vi "Options GUI.vi"(7 "Initial Tab(0)":i32, 11 "error in (no error)":errorcluster) -> (8 "OK":bool, 14 "Restart software":bool, 15 "error out":errorcluster)   [LabVIEW 2011]
uses:
  Options Page 1 for display.ctl
  Options Page 2.ctl
  Options Page 6 (Err).ctl
  Options Page 7 (Expert).ctl
  GUI/Options/Modem simulation setup.ctl
  Options Page 3.ctl
  PCP interface/PCP type List.ctl
  PCP interface/PSU Type.ctl
  Options Page 4.ctl
  Tool/Stroke force selector.ctl
  Tool/Default anchor behavior.ctl
  Tool/Default stroker behavior.ctl
  GUI/Controls/Slips Type Radio.ctl
  Options Page 5.ctl
  Options Page 8 (Depth).ctl
  Action GFV Settings.ctl
  Options PageID.ctl
  <vilib>/Utility/libraryn.llb/Check if File or Folder Exists.vi
panel:
  in  "Help":bool
  in  "Create system report":bool
  in  "Cancel":bool
  in  "OK btn":bool
  in  "Tab Control":T1(tab)
  in  "Modem Status":u16(ring) items=["Select Port", "COM19", "Refresh"]
  in  "Tractor Interface":u16(ring) items=["Select Port", "COM19", "Refresh"]
  in  "Modem Data":u16(ring) items=["Select Port", "COM19", "Refresh"]
  in  "Power Supply/PCP":u16(ring) items=["Select Port", "COM19", "Refresh"]
  in  "P 1 (App)":T2
  in  "Power supply connected":string
  in  "P 3":T3={"Min resistance"=40.0, "Max resistance"=70.0, "Head voltage range"=enum."0 - 450V", "Max voltage jump"=10.0, "Maximum resistance change"=2.0, "Start Telemetry Voltage"=35.0, "Start Telemetry Timeout"=20.0, "Start Motor Voltage"=160.0, "Stop Motor Voltage"=1.0, "Pass Mode Warning Voltage"=1.0, "Relay Switch Voltage"=160.0, "Relay Status Loss Voltage"=0.0, "Samples to average"=1, "PSU type DO NOT USE"=enum."Magna 8.3A", "Magna OVP"=1.0, "Magna Current Limit"=160.0} {"Relay Status Loss Voltage" min=0.0 max=500.0 format="%#.0f"; "Relay Switch Voltage" min=5.0 max=500.0 format="%#.0f"; "Magna Current Limit" min=0.0 max=20.0 format="%.1f"; "Magna OVP" min=0.0 max=1500.0 format="%#.0f"; "Pass Mode Warning Voltage" min=5.0 max=500.0 format="%#.0f"; "Stop Motor Voltage" min=5.0 max=500.0 format="%#.0f"; "Start Telemetry Timeout" min=0.0 max=500.0 format="%#.0f"; "Samples to average" min=1 max=10; "Start Motor Voltage" min=5.0 max=500.0 format="%#.0f"; "Start Telemetry Voltage" min=5.0 max=500.0 format="%#.0f"; "Maximum resistance change" min=1.0 max=100.0 format="%#.0f"; "Max voltage jump" min=5.0 max=500.0 format="%#.0f"; "Max resistance" min=30.0 max=500.0 format="%#.0f"; "Min resistance" min=0.0 max=500.0 format="%#.0f"}
  out "Force Unit 2":string
  out "Force Unit":string
  in  "P 4":T6={"Solenoid & Relay latching time"=40, "Stroker relay 1"=1.0, "Stroker Relay 2"=40.0, "Stroker Solenoid limit"=0.0, "Force det."=enum."Stroke in = node 1", "Stroke force lim."=0.0, "Anchor Enabled Pressure"=0.05, "Tacometer puls"=0.3, "Default anchor behavior"=enum."Do nothing", "Default stroker behavior"=enum."Do nothing", "Default stroker force limit (tonne)"=0.0, "Slips Size"=enum."338 MRS"} {"Default stroker force limit (tonne)" format="%.2f"; "Stroker Relay 2" format="%.2f"; "Stroker relay 1" format="%.2f"; "Tacometer puls" format="%.2f"; "Anchor Enabled Pressure" format="%.2f"; "Stroke force lim." format="%.2f"; "Stroker Solenoid limit" format="%.2f"}
  in  "P 5":T11={"Solenoid & Relay latching time"=0, "Driller relay 1"=0.3, "Driller Relay 2"=0.2, "Driller  Solenoid limit"=0.2} {"Driller  Solenoid limit" format="%.2f"; "Driller Relay 2" format="%.2f"; "Driller relay 1" format="%.2f"}
  in  "P 2":T12={"Solenoid & Relay latching time"=0, "Tractor relay 1"=0.3, "Tractor relay 2"=0.2, "Tractor Solenoid limit"=0.2} {"Tractor Solenoid limit" format="%.2f"; "Tractor relay 2" format="%.2f"; "Tractor relay 1" format="%.2f"}
  in  "P 6 (Err)":T13
  in  "P 7 (Expert)":T14={"Show Debug"=FALSE, "Log debug messages"=FALSE, "Additional debug messages"=FALSE, "Start Beagle with Simulator data"=FALSE, "Workshop mode"=FALSE, "Modem baud"=38400, "enumCANCOM"=FALSE, "Modem sim"={"Modem dealay sim"=FALSE, "Sim baud Tx"=1200, "Bit Error fraction Tx"=0.0, "Sim baud Rx"=1200, "Bit Error fraction Rx"=0.0}, "Telemetry Timeout Disable"=20, "Buffer size"=20, "Upd regular data"=FALSE, "Cable comp"={"VMOD1 Voltage(V)"=1.0, "VMOD2 Voltage(V)"=8.0}} {"Cable comp"."VMOD2 Voltage(V)" format="%.1f"; "Cable comp"."VMOD1 Voltage(V)" format="%.1f"; "Telemetry Timeout Disable" min=2 max=20 step=2; "Modem baud" items=["38400 (Normal use)"=38400, "9600 (Development)"=9600]; "Modem sim"."Bit Error fraction Rx" format="%.9f"; "Modem sim"."Sim baud Rx" items=["9600"=9600, "4800"=4800, "2400"=2400, "1200"=1200, "1000"=1000, "800"=800, "600"=600, "400"=400, "200"=200]; "Modem sim"."Bit Error fraction Tx" format="%.9f"; "Modem sim"."Sim baud Tx" items=["9600"=9600, "4800"=4800, "2400"=2400, "1200"=1200, "1000"=1000, "800"=800, "600"=600, "400"=400, "200"=200]; "Buffer size" min=86400 max=1209600}
  in  "Set current depth":bool caption="Solonoid 3 off"
  in  "P 8 (Depth)":T16={"Winch Spool Circumference"=100.0, "Winch Pulses per Revolution"=160.0, "Current Depth"=100.0} {"Current Depth" format="%#.7f"; "Winch Pulses per Revolution" min=1.0 max=100000.0 step=1.0 format="%#.0f"; "Winch Spool Circumference" min=0.0 max=200.0 format="%#.7f"}
  # "Tab header s can be changed as wanted\n\nCustom can be used for completly ccutom behavior,\nmust then highjack  an other hidden page, for settings"
  # "Add custom behavior taht cvan not be replicated by a simple cluster with valisdity checking"
  # "* Changes to marked options will take effect the next time you start Beagle."
  # "Ohm"
  # "Ohm"
  # "V"
  # "Ohm"
  # "V"
  # "s"
  # "V"
  # "V"
  # "V"
  # "V"
  # "V"
  # "ms"
  # "When both relays are used in \nthe same operation, the lowest\nlimit is used for both."
  # "A"
  # "A"
  # "A"
  # "Bar"
  # "ms"
  # "When both relays are used in \nthe same operation, the lowest\nlimit is used for both."
  # "A"
  # "A"
  # "A"
  # "ms"
  # "When both relays are used in \nthe same operation, the lowest\nlimit is used for both."
  # "A"
  # "A"
  # "A"
  # "Add custom behavior taht cvan not be replicated by a simple cluster with valisdity checking"
  # "Hide this page, remove this button\nAdd custom behavior if needed, using this excample"
  # "Add custom behavior taht cvan not be replicated by a simple cluster with valisdity checking"
  # "m"
  # "Pulses"
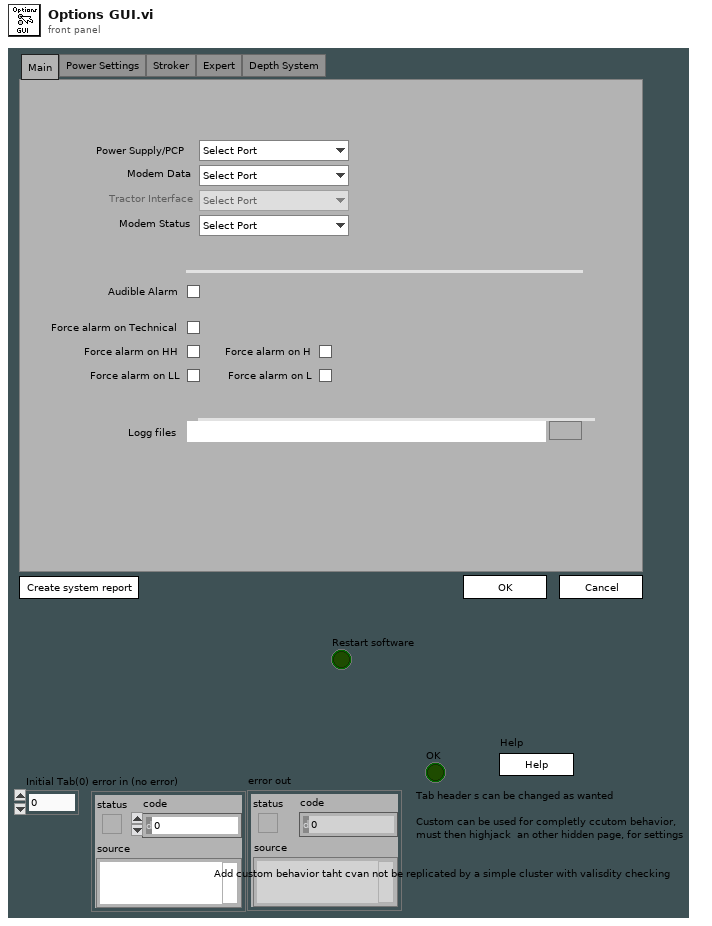
[diagram p1: front panel]
types:
  T1 = enum32{"Main", "Power Settings", "Stroker", "Driller", "Tractor", "Custom 1", "Custom 2", "Error and Events", "Expert", "Depth System"}
  T2 = typedef "Options Page 1 for display.ctl" = cluster{"Logg files":path, "Audible Alarm":bool, "Force alarm on Technical":bool, "Force alarm on HH":bool, "Force alarm on LL":bool, "Force alarm on H":bool, "Force alarm on L":bool}
  T3 = typedef "Options Page 3.ctl" = cluster{"Min resistance":dbl, "Max resistance":dbl, "Head voltage range":T4, "Max voltage jump":dbl, "Maximum resistance change":dbl, "Start Telemetry Voltage":dbl, "Start Telemetry Timeout":dbl, "Start Motor Voltage":dbl, "Stop Motor Voltage":dbl, "Pass Mode Warning Voltage":dbl, "Relay Switch Voltage":dbl, "Relay Status Loss Voltage":dbl, "Samples to average":i32, "PSU type DO NOT USE":T5, "Magna OVP":dbl, "Magna Current Limit":dbl}
  T4 = typedef "PCP type List.ctl" = enum16{"0 - 350V", "0 - 450V", "0 - 600V"}
  T5 = typedef "PSU Type.ctl" = enum16{"Unipower", "Magna 8.3A", "Magna 12A", "None"}
  T6 = typedef "Options Page 4.ctl" = cluster{"Solenoid & Relay latching time":u16, "Stroker relay 1":dbl, "Stroker Relay 2":dbl, "Stroker Solenoid limit":dbl, "Force det.":T7, "Stroke force lim.":dbl, "Anchor Enabled Pressure":dbl, "Tacometer puls":dbl, "Default anchor behavior":T8, "Default stroker behavior":T9, "Default stroker force limit (tonne)":dbl, "Slips Size":T10}
  T7 = typedef "Stroke force selector.ctl" = enum16{"Stroke in = node 1", "Strok out = node 1"}
  T8 = typedef "Default anchor behavior.ctl" = enum16{"Do nothing", "Set Anchor", "Release Anchor"}
  T9 = typedef "Default stroker behavior.ctl" = enum16{"Do nothing", "Stop", "Go Out", "Go In"}
  T10 = typedef "Slips Type Radio.ctl" = enum32{"No Selection", "338 MRS", "3,9 MRS"}
  T11 = typedef "Options Page 5.ctl" = cluster{"Solenoid & Relay latching time":u16, "Driller relay 1":dbl, "Driller Relay 2":dbl, "Driller  Solenoid limit":dbl}
  T12 = typedef "Options Page 2.ctl" = cluster{"Solenoid & Relay latching time":u16, "Tractor relay 1":dbl, "Tractor relay 2":dbl, "Tractor Solenoid limit":dbl}
  T13 = typedef "Options Page 6 (Err).ctl" = cluster{"Error and event files":path}
  T14 = typedef "Options Page 7 (Expert).ctl" = cluster{"Show Debug":bool, "Log debug messages":bool, "Additional debug messages":bool, "Start Beagle with Simulator data":bool, "Workshop mode":bool, "Modem baud":u16, "enumCANCOM":bool, "Modem sim":T15, "Telemetry Timeout Disable":i32, "Buffer size":i32, "Upd regular data":bool, "Cable comp":cluster{"VMOD1 Voltage(V)":dbl, "VMOD2 Voltage(V)":dbl}}
  T15 = typedef "Modem simulation setup.ctl" = cluster{"Modem dealay sim":bool, "Sim baud Tx":u16, "Bit Error fraction Tx":dbl, "Sim baud Rx":u16, "Bit Error fraction Rx":dbl}
  T16 = typedef "Options Page 8 (Depth).ctl" = cluster{"Winch Spool Circumference":dbl, "Winch Pulses per Revolution":dbl, "Current Depth":dbl}
  T17 = typedef "Action GFV Settings.ctl" = enum16{"Init", "Get From INI", "Put In INI", "Get Settings", "Get Update Index", "Set Setting"}
  T18 = typedef "Options  All pages and custom.ctl" = cluster{"P 1 (App)":T19, "P 2":T12, "P 3":T3, "P 4":T6, "P 5":T11, "P 6 (Err)":T13, "P 7 (Expert)":T14, "P 8 (Depth)":T16, "C 1":T20, "C 2":T21}
  T19 = typedef "Options Page 1 (App).ctl" = cluster{"Result files":path, "PCP Interface":string, "Tractor/Stroker Interface":string, "Tractor Interface":string, "Modem Status Interface":string, "Audible Alarm":bool, "Force alarm on Technical":bool, "Force alarm on HH":bool, "Force alarm on LL":bool, "Force alarm on H":bool, "Force alarm on L":bool}
  T20 = typedef "Options Custom 1.ctl" = cluster{"Depth Updated":bool, "Depth Offset":dbl}
  T21 = typedef "Options Custom 2.ctl" = cluster{"Placeholder":bool}
  T22 = enum8{"Enabled", "Disabled", "Disabled and Grayed Out"}
  T23 = typedef "List of tools.ctl" = enum16{"Stroker", "Driller", "Tractor"}
  T24 = typedef "User Indikator.ctl" = cluster{"User Name":string, "Super User":T25}
  T25 = typedef "Super User bool indikator.ctl" = bool
  T26 = typedef "Options PageID.ctl" = enum16{"P 1 (App)", "P 2", "P 3", "P 4", "P 5", "P 6 (Err)", "P 7 (Expert)", "P 8", "C 1", "C 2"}
  T27 = enum16{"open", "replace", "create", "open or create", "replace or create", "replace or create with confirmation"}
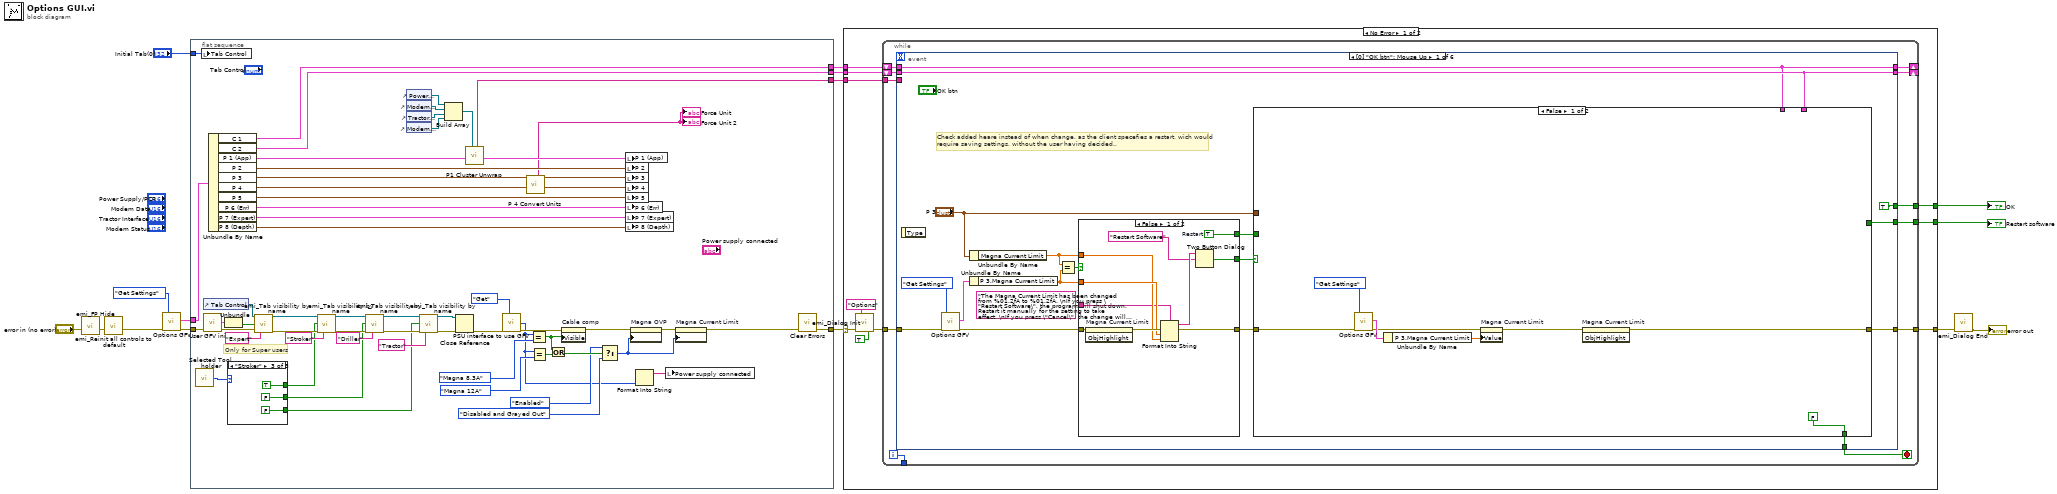
[diagram p0: block diagram]
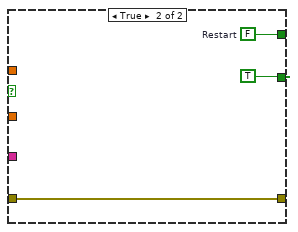
[diagram p2: hidden frame]
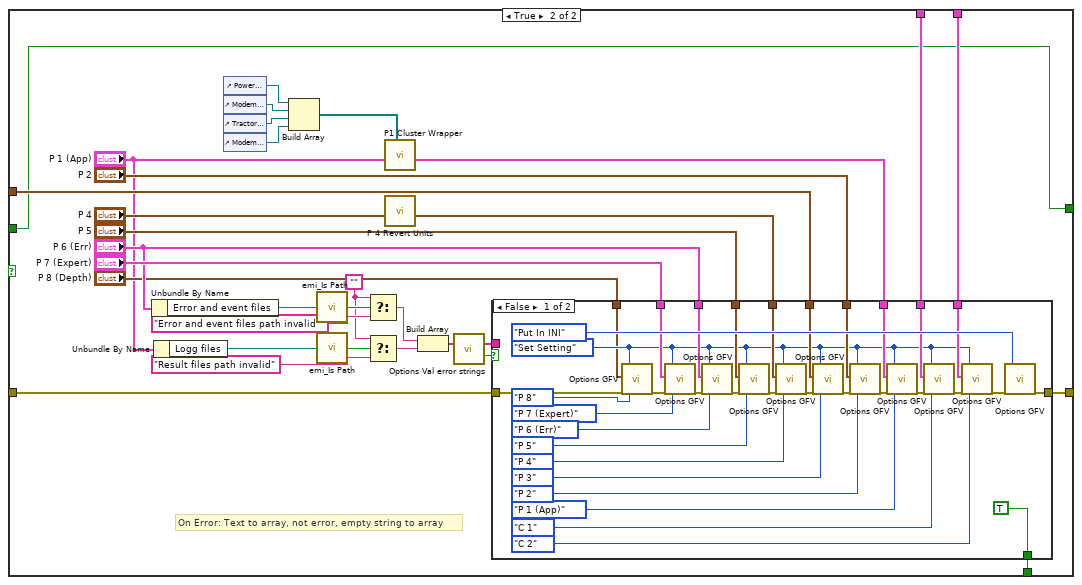
[diagram p3: hidden frame]
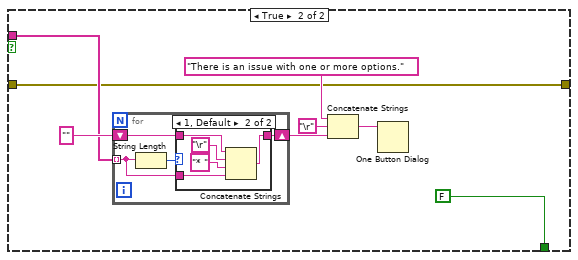
[diagram p4: hidden frame]
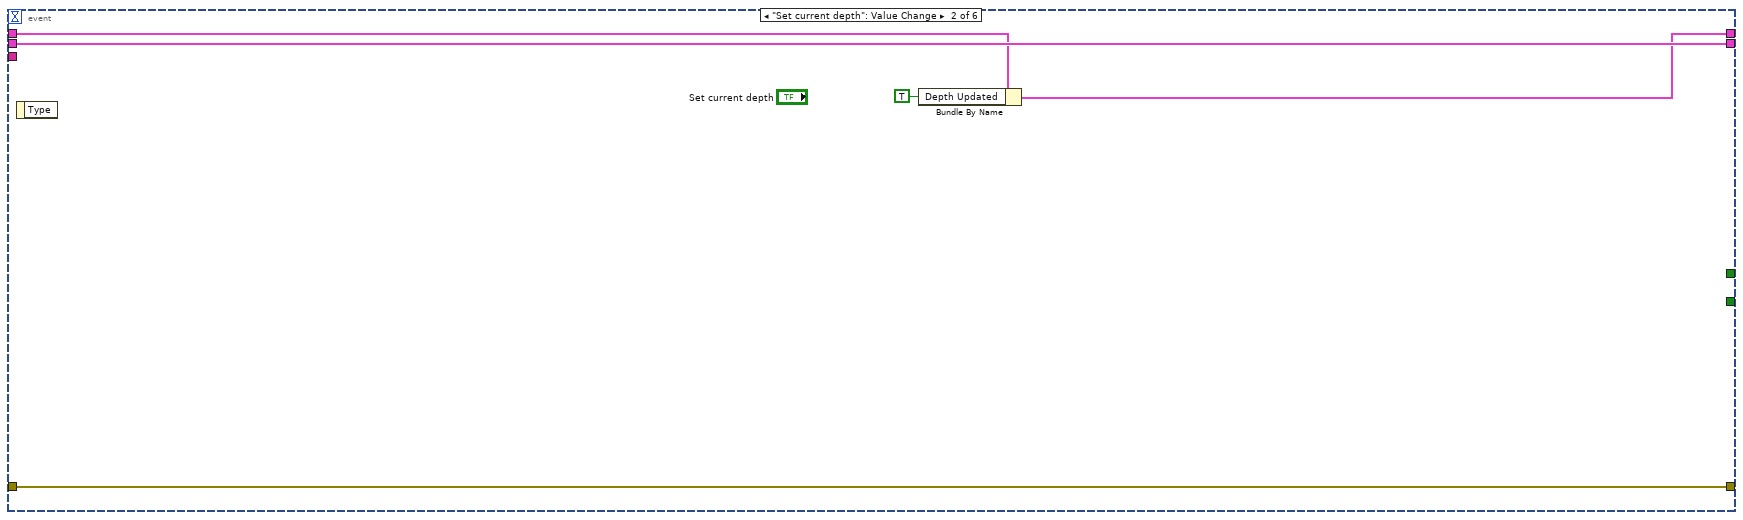
[diagram p6: hidden frame]
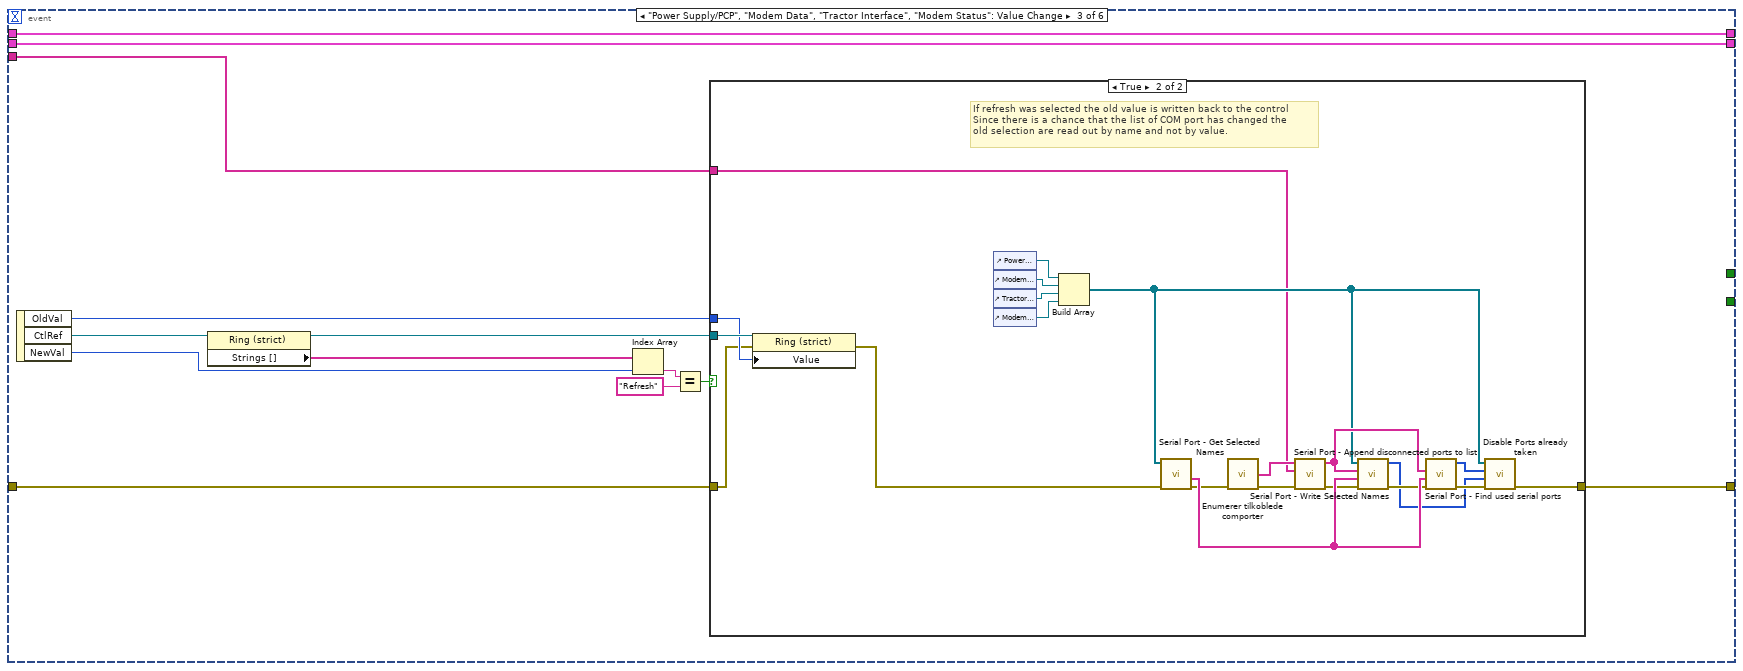
[diagram p7: hidden frame]
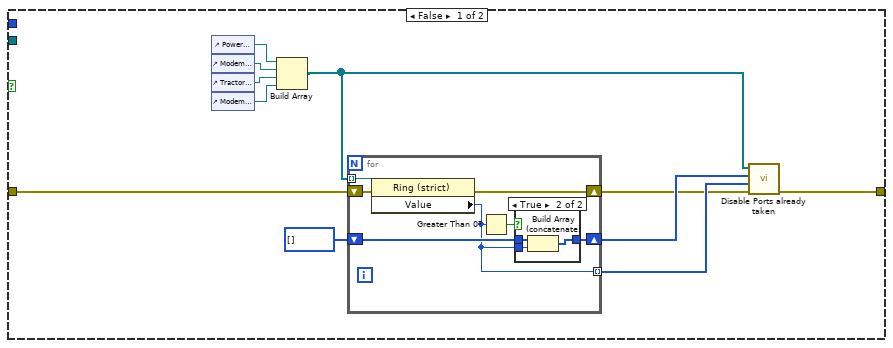
[diagram p8: hidden frame]
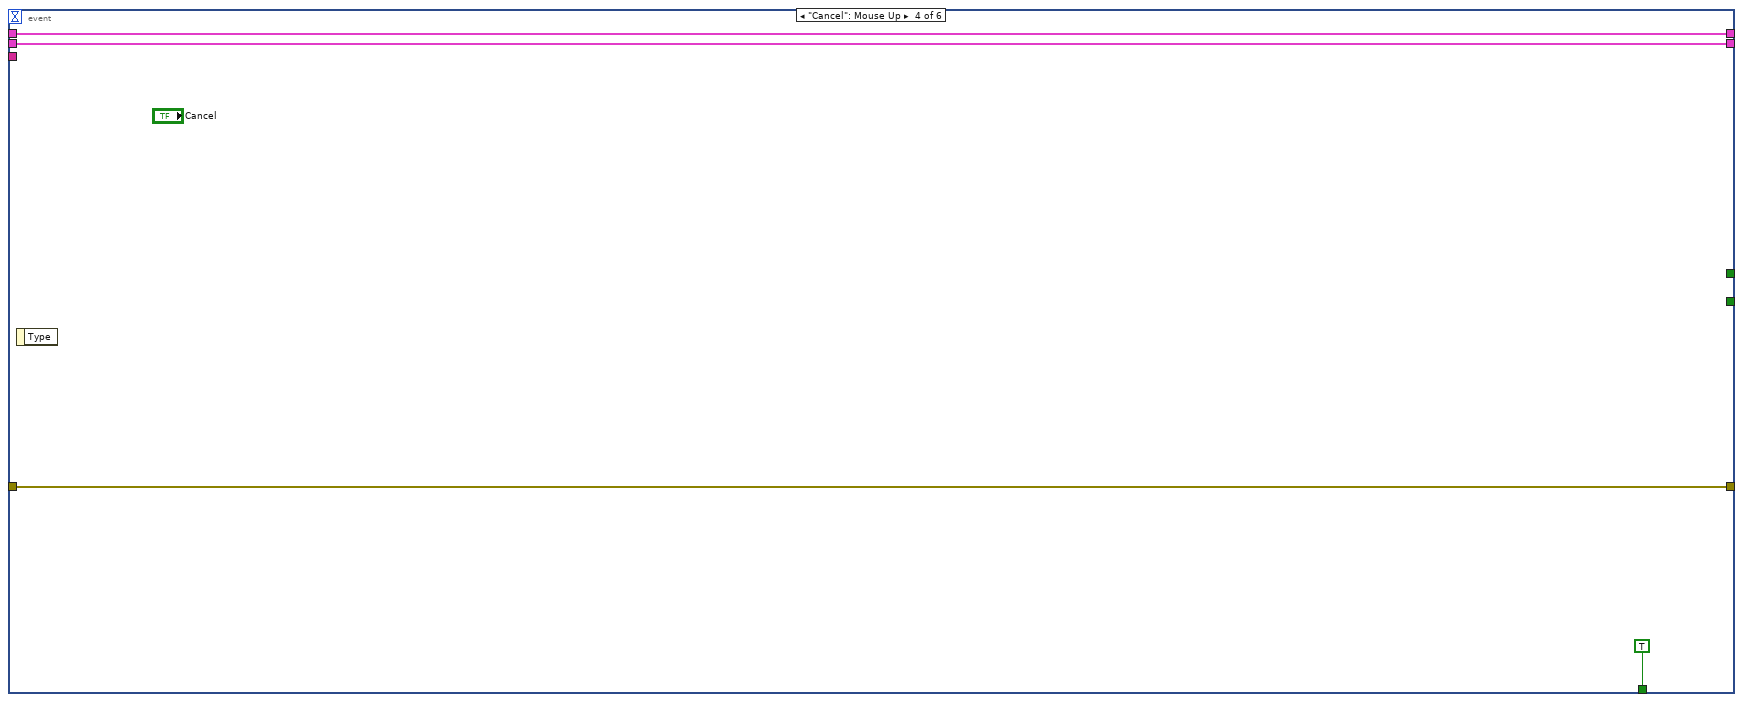
[diagram p10: hidden frame]
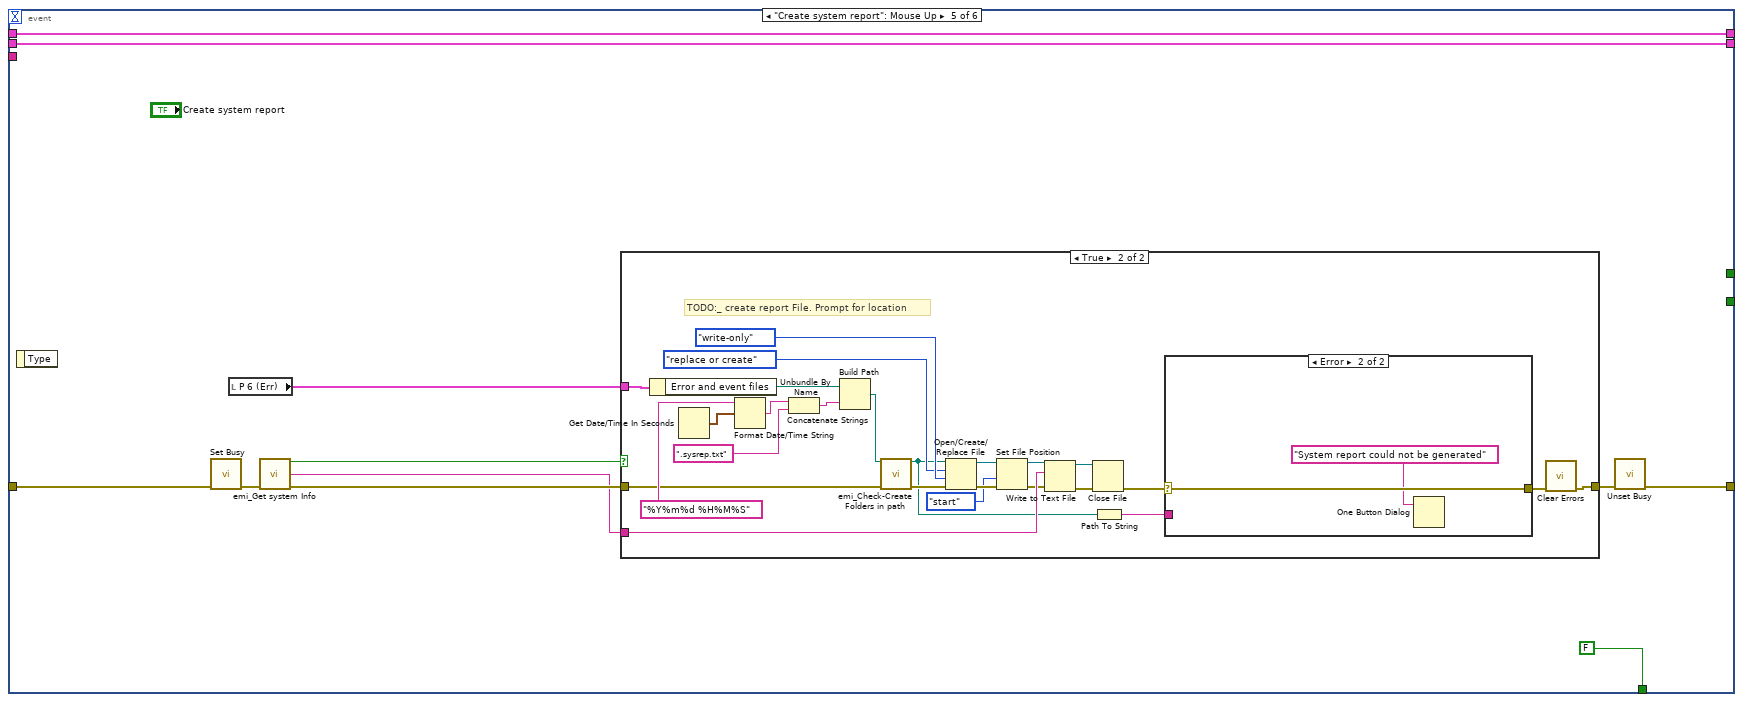
[diagram p11: hidden frame]
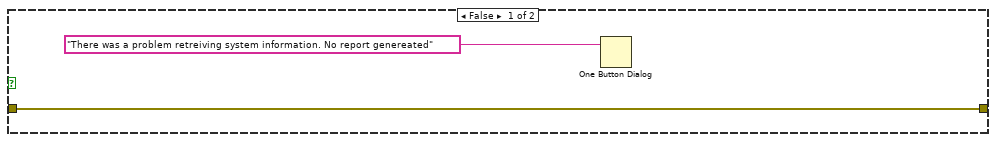
[diagram p12: hidden frame]
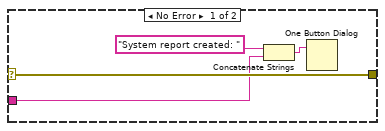
[diagram p13: hidden frame]
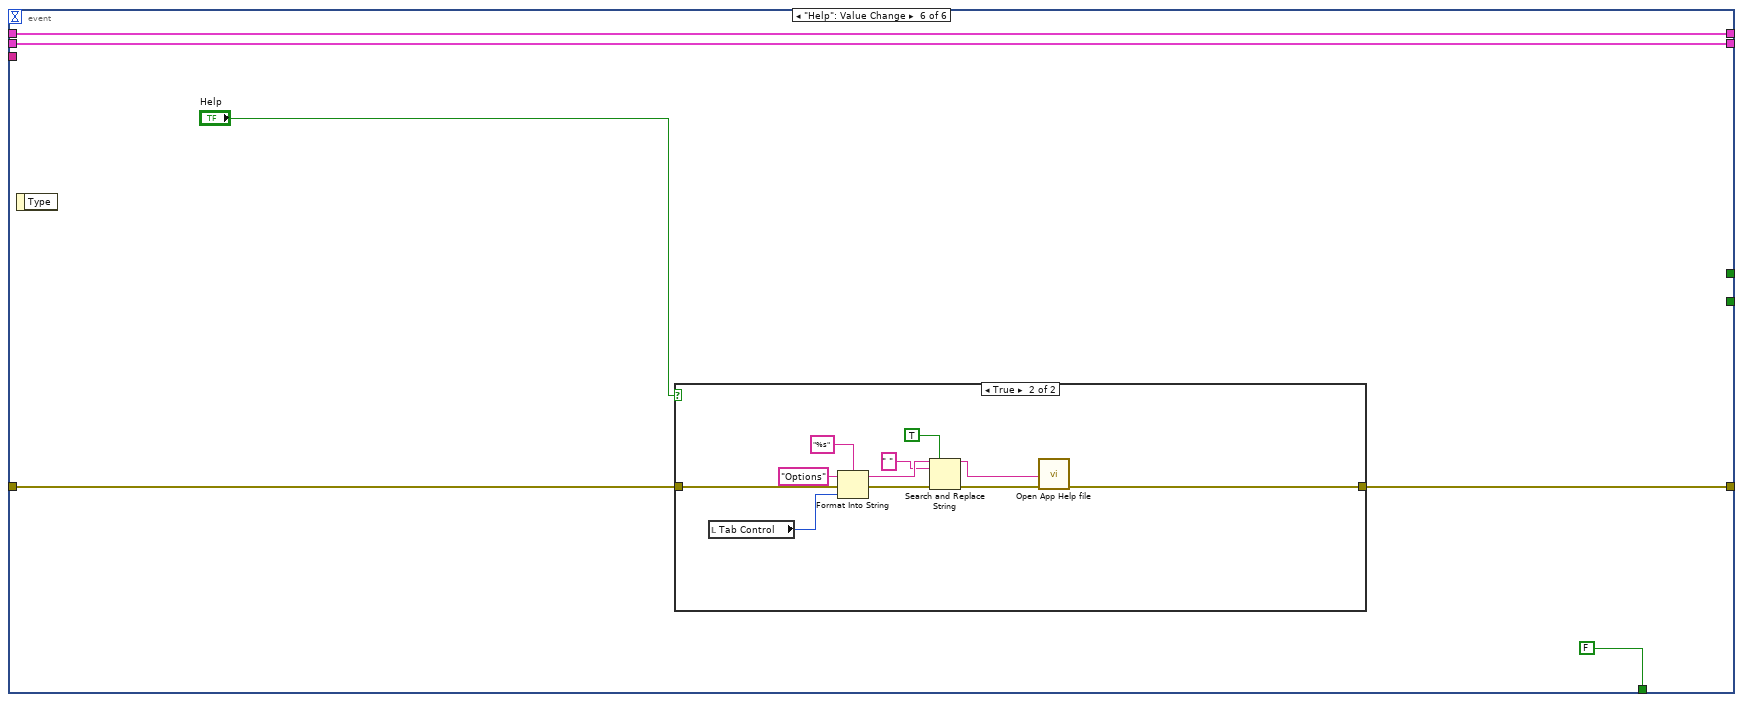
[diagram p14: hidden frame]
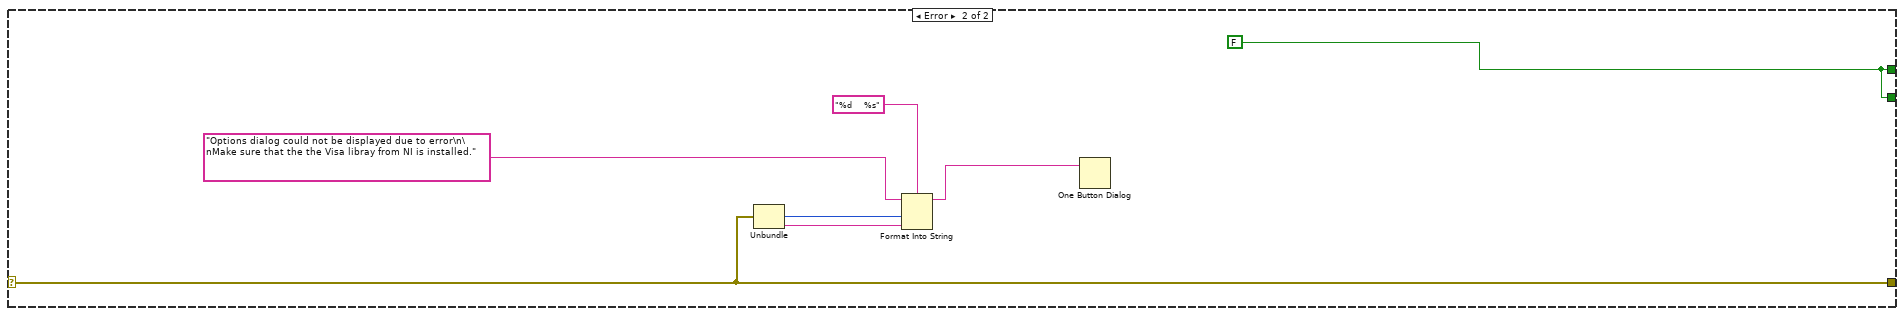
[diagram p16: hidden frame]
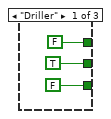
[diagram p17: hidden frame]
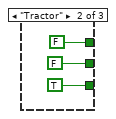
[diagram p18: hidden frame]
diagram:
  n1 = call "emi_FP Hide.vi"("error in (no error)"="error in (no error)") -> ("error out"=w5:errorcluster)  [unwired: 13 in, 1 out]
  n2 = call "emi_Reinit all controls to default.vi"("error in (no error)"=w5) -> ("error out"=w4:errorcluster)  [unwired: 13 in, 1 out]
  n3 = call "Options GFV.vi"("error in (no error)"=w4, "Action(Get Settings)"=Action_GFV_Settings."Get Settings" ("Action")) -> ("Options"=w12:T18, "error out"=w13:errorcluster)  [unwired: 15 in, 1 out]
  n4 = flat-sequence {
    tunnel: [w28] -> w3
    tunnel: "Initial Tab(0)" -> [w70]
    tunnel: w13 -> [w68]
    tunnel: w12 -> [w69]
    tunnel: [w45] -> w9
    tunnel: [w46] -> w10
    tunnel: [w33] -> w2
    frame #0 {
      # "Only for Super users"
      n5 = call "Selected Tool holder.vi"() -> ("Tool out"=w51:T23)  [unwired: 14 in, 1 out]
      n6 = local write "Tab Control"(w70) -> ()
      n7 = control-ref of="Tab Control"() -> (w65:refnum<vi>)
      n8 = call "User GFV ini.vi"("error in (no error)"=w68) -> ("User ID out"=w67:T24, "error out"=w66:errorcluster)  [unwired: 13 in]
      n9 = Unbundle By Name(w69) -> ("C 1"=w46:T20, "C 2"=w45:T21, "P 1 (App)"=w36:T19, "P 2"=w74:T12, "P 3"=w73:T3, "P 4"=w43:T6, "P 5"=w47:T11, "P 6 (Err)"=w72:T13, "P 7 (Expert)"=w71:T14, "P 8 (Depth)"=w44:T16)
      n10 = Unbundle(w67) -> ("Super User"=w64:T25)  [unwired: 1 out]
      n11 = case shown="\"Stroker\"" w51 {
        tunnel: [FALSE ("Visibil(T)") FALSE ("Visibil(T)") TRUE ("Visibil(T)")] -> w50
        tunnel: [TRUE ("Visibil(T)") FALSE ("Visibil(T)") FALSE ("Visibil(T)")] -> w49
        tunnel: [FALSE ("Visibil(T)") TRUE ("Visibil(T)") FALSE ("Visibil(T)")] -> w48
        frame "Driller" {
        }
        frame "Tractor" {
        }
        frame "Stroker" {
        }
      }
      n12 = call "emi_Tab visibility by name.vi"("reference"=w65, "Visibil(T)"=w64, "error in (no error)"=w66, "Tab name(\"Debug\")"="Expert" ("Tab name(\"Debug\")")) -> ("reference out"=w61:refnum<vi>, "error out"=w62:errorcluster)  [unwired: 10 in]
      n13 = call "emi_Tab visibility by name.vi"("reference"=w61, "Visibil(T)"=w50, "error in (no error)"=w62, "Tab name(\"Debug\")"="Stroker" ("Tab name(\"Debug\")")) -> ("reference out"=w59:refnum<vi>, "error out"=w60:errorcluster)  [unwired: 10 in]
      n14 = call "emi_Tab visibility by name.vi"("reference"=w59, "Visibil(T)"=w49, "error in (no error)"=w60, "Tab name(\"Debug\")"="Driller" ("Tab name(\"Debug\")")) -> ("reference out"=w57:refnum<vi>, "error out"=w58:errorcluster)  [unwired: 10 in]
      n15 = control-ref of="Power Supply/PCP"() -> (w41:refnum<vi>)
      n16 = control-ref of="Modem Data"() -> (w40:refnum<vi>)
      n17 = control-ref of="Tractor Interface"() -> (w39:refnum<vi>)
      n18 = control-ref of="Modem Status"() -> (w38:refnum<vi>)
      n19 = call "emi_Tab visibility by name.vi"("reference"=w57, "Visibil(T)"=w48, "error in (no error)"=w58, "Tab name(\"Debug\")"="Tractor" ("Tab name(\"Debug\")")) -> ("reference out"=w55:refnum<vi>, "error out"=w56:errorcluster)  [unwired: 10 in]
      n20 = Build Array(w41, w40, w39, w38) -> (w35:refnum<vi>[])
      n21 = Close Reference(reference=w55, error in (no error)=w56) -> (error out=w32:errorcluster)
      n22 = call "P1 Cluster Unwrap.vi"("COM Selector Refs"=w35, "P 1 (App) in"=w36) -> ("P 1 (App) out"=w37:T2, "Initial selection"=w33:string[])  [unwired: 8 in]
      n23 = call "PSU interface to use GFV.vi"("Action"=enum16{"Get", "Set"}."Get", "error in (no error)"=w32) -> ("PSU type  out"=w17:T5, "error out"=w30:errorcluster)  [unwired: 12 in]
      n24 = call "P 4 Convert Units.vi"("P 4"=w43) -> ("P 4"=w42:T6, "Unit"=→"Force Unit" →"Force Unit 2":string)  [unwired: 9 in]
      n25 = Equal?(x=w17, y=PSU_Type."Magna 8.3A") -> (x = y?=w25:bool)
      n26 = Equal?(x=w17, y=PSU_Type."Magna 12A") -> (x = y?=w26:bool)
      n27 = Or(x=w25, y=w26) -> (x .or. y?=w21:bool)
      n28 = property on="Cable comp" class="Clust (strict)"(error in=w30, "Visible"=w25) -> (error out=w24:errorcluster)  [unwired: 1 in, 1 out]
      n29 = Select(t=T22."Enabled" ("Disabled"), s=w21, f=T22."Disabled and Grayed Out" ("Disabled")) -> (s? t:f=w18:T22)
      n30 = local write "P 1 (App)"(w37) -> ()
      n31 = local write "P 2"(w74) -> ()
      n32 = local write "P 3"(w73) -> ()
      n33 = local write "P 4"(w42) -> ()
      n34 = local write "P 5"(w47) -> ()
      n35 = local write "P 6 (Err)"(w72) -> ()
      n36 = local write "P 7 (Expert)"(w71) -> ()
      n37 = local write "P 8 (Depth)"(w44) -> ()
      n38 = property on="Magna OVP" class="DigNum (strict)"(error in=w24, "DisabledEnum"=w18) -> (error out=w23:errorcluster)  [unwired: 1 in, 1 out]
      n39 = Format Into String(w17) -> (resulting string=w16:string)  [unwired: 3 in, 1 out]
      n40 = local write "Power supply connected"(w16) -> ()
      n41 = property on="Magna Current Limit" class="DigNum (strict)"(error in=w23, "DisabledEnum"=w18) -> (error out=w22:errorcluster)  [unwired: 1 in, 1 out]
      n42 = call <vilib>:"Clear Errors.vi"("error in (no error)"=w22) -> ("error out"=w28:errorcluster)  [unwired: 6 in]
    }
  }
  n43 = case shown="No Error" w3 {
    selector: w3 -> [w86 w363]
    tunnel: w10 -> [w93 _]
    tunnel: w9 -> [w92 _]
    tunnel: [w91 w357] -> w8
    tunnel: [w90 w363] -> w7
    tunnel: w2 -> [w85 _]
    tunnel: [w84 w357] -> w1
    frame No Error {
      n44 = call "emi_Dialog Init.vi"("Header String(\"\")"="Options" ("Header String(\"\")"), "error in"=w86, "Modal(T)"=TRUE) -> ("error out"=w89:errorcluster)  [unwired: 12 in]
      n45 = while {
        tunnel: [w104] -> _
        tunnel: w89 -> [w103]
        tunnel: [w102] -> w90
        shift-right: [w99] -> _
        shift-left: w93 -> [w101]
        shift-right: [w98] -> _
        shift-left: w92 -> [w100]
        tunnel: [w97] -> w91
        tunnel: w85 -> [w95]
        tunnel: [w94] -> w84
        i -> [w104]
        stop <- w96 stop-if-true
        n46 = event shown="[0] \"OK btn\": Mouse Up" {
          selector: _ -> [_ _ _ _ _ _]
          dyn-events: _ -> [_ _ _ _ _ _]
          timeout: _ -> [_ _ _ _ _ _]
          tunnel: [w122 _ _ TRUE FALSE FALSE] -> w96
          tunnel: w103 -> [w117 w234 w245 w293 w304 w340]
          tunnel: [w121 w234 w244 w293 w303 w341] -> w102
          tunnel: w101 -> [w118 w232 w247 w292 w296 w343]
          tunnel: w100 -> [w120 w233 w246 w291 w295 w342]
          tunnel: [w118 w231 w247 w292 w296 w343] -> w99
          tunnel: [w120 w233 w246 w291 w295 w342] -> w98
          tunnel: [TRUE _ _ _ _ _] -> w97
          tunnel: w95 -> [_ _ w235 _ _ _]
          tunnel: [w105 _ _ _ _ _] -> w94
          event "OK btn": Mouse Up {
            # "Check added heare instead of when change, as the client specefies a restart, wich would \nrequire saving settings, without the user having decided.,"
            n47 = event-data() -> ()  [unwired: 1 in, 1 out]
            n48 = call "Options GFV.vi"("error in (no error)"=w117, "Action(Get Settings)"=Action_GFV_Settings."Get Settings") -> ("Options"=w114:T18, "error out"=w111:errorcluster)  [unwired: 15 in, 1 out]
            n49 = Unbundle By Name("P 3") -> ("Magna Current Limit"=w108:dbl)
            n50 = Unbundle By Name(w114) -> ("P 3.Magna Current Limit"=w109:dbl)
            n51 = Equal?(x=w108, y=w109) -> (x = y?=w113:bool)
            n52 = case shown="False" w113 {
              tunnel: [w124 TRUE] -> w112
              tunnel: w111 -> [w132 w134]
              tunnel: [w130 w134] -> w110
              tunnel: w109 -> [w129 _]
              tunnel: w108 -> [w128 _]
              tunnel: "The Magna Current Limit has been changed from %01.2fA to %01.2fA. \nIf you press \"Restart Software\", the program will shut down. Restart it manually for the setting to take effect. \nIf you press \"Cancel\", the change will be reverted." ("format string") -> [w127 _]
              tunnel: [w123 w133] -> w106
              frame False {
                w123 = TRUE  # Restart
                n53 = invoke on="Magna Current Limit" class="DigNum (strict)" method="ObjHighlight"(error in=w132) -> (error out=w131:errorcluster)  [unwired: 2 in, 2 out]
                n54 = Format Into String(format string=w127, error in=w131, w129, w128) -> (resulting string=w126:string, error out=w130:errorcluster)  [unwired: 1 in]
                n55 = Two Button Dialog(message=w126, 2:"Restart Software" ("T button name (\"OK\")")) -> (T button?=w124:bool)  [unwired: 1 in]
              }
              frame True {
                w133 = FALSE  # Restart
              }
            }
            n56 = case shown="False" w112 {
              tunnel: [FALSE w176] -> w122
              tunnel: [w136 w175] -> w121
              tunnel: "P 3" -> [_ w174]
              tunnel: w110 -> [w140 w170]
              tunnel: w120 -> [_ w156]
              tunnel: w118 -> [_ w154]
              tunnel: w106 -> [_ w144]
              tunnel: [_ w144] -> w105
              frame False {
                n57 = call "Options GFV.vi"("error in (no error)"=w140, "Action(Get Settings)"=Action_GFV_Settings."Get Settings") -> ("Options"=w142:T18, "error out"=w138:errorcluster)  [unwired: 15 in, 1 out]
                n58 = Unbundle By Name(w142) -> ("P 3.Magna Current Limit"=w139:dbl)
                n59 = property on="Magna Current Limit" class="DigNum (strict)"(error in=w138, "Value"=w139) -> (error out=w137:errorcluster)  [unwired: 1 in, 1 out]
                n60 = invoke on="Magna Current Limit" class="DigNum (strict)" method="ObjHighlight"(error in=w137) -> (error out=w136:errorcluster)  [unwired: 2 in, 2 out]
              }
              frame True {
                w160 = ""
                # "On Error: Text to array, not error, empty string to array"
                n61 = Unbundle By Name("P 6 (Err)") -> ("Error and event files"=w166:path)
                n62 = Unbundle By Name("P 1 (App)") -> ("Logg files"=w165:path)
                n63 = control-ref of="Power Supply/PCP"() -> (w146:refnum<vi>)
                n64 = control-ref of="Modem Data"() -> (w147:refnum<vi>)
                n65 = control-ref of="Tractor Interface"() -> (w148:refnum<vi>)
                n66 = control-ref of="Modem Status"() -> (w149:refnum<vi>)
                n67 = Build Array(w146, w147, w148, w149) -> (w145:refnum<vi>[])
                n68 = call "emi_Is Path.vi"("Path"=w166) -> ("Path?"=w164:bool)  [unwired: 14 in]
                n69 = call "emi_Is Path.vi"("Path"=w165) -> ("Path?"=w163:bool)  [unwired: 14 in]
                n70 = Select(t=w160, s=w164, f="Error and event files path invalid") -> (s? t:f=w158:string)
                n71 = Select(t=w160, s=w163, f="Result files path invalid") -> (s? t:f=w157:string)
                n72 = call "P1 Cluster Wrapper.vi"("COM Selector Refs"=w145, "P 1 (App) in"="P 1 (App)") -> ("P 1 (App) out"=w150:T19)  [unwired: 8 in, 1 out]
                n73 = call "P 4 Revert Units.vi"("P 4"="P 4") -> ("P 4"=w152:T6)  [unwired: 10 in]
                n74 = Build Array(w158, w157) -> (w159:string[])
                n75 = call "Options Val error strings.vi"("Array of error strings"=w159) -> ("Array of error strings out"=w171:string[], "Error"=w172:bool)  [unwired: 13 in]
                n76 = case shown="False" w172 {
                  tunnel: [TRUE FALSE] -> w176
                  tunnel: [w204 w212] -> w175
                  tunnel: w150 -> [w196 _]
                  tunnel: "P 2" -> [w195 _]
                  tunnel: w174 -> [w194 _]
                  tunnel: w152 -> [w193 _]
                  tunnel: "P 5" -> [w192 _]
                  tunnel: "P 6 (Err)" -> [w191 _]
                  tunnel: "P 7 (Expert)" -> [w190 _]
                  tunnel: w171 -> [_ w213]
                  tunnel: w170 -> [w181 w212]
                  tunnel: w156 -> [w185 _]
                  tunnel: w154 -> [w186 _]
                  tunnel: "P 8 (Depth)" -> [w177 _]
                  frame False {
                    w179 = Action_GFV_Settings."Set Setting" ("Action")
                    n77 = call "Options GFV.vi"("Anything"=w177, "error in (no error)"=w181, "Action(Get Settings)"=w179, "Setting ID"=Options_PageID."P 8") -> ("error out"=w180:errorcluster)  [unwired: 13 in, 2 out]
                    n78 = call "Options GFV.vi"("Anything"=w190, "error in (no error)"=w180, "Action(Get Settings)"=w179, "Setting ID"=Options_PageID."P 7 (Expert)") -> ("error out"=w208:errorcluster)  [unwired: 13 in, 2 out]
                    n79 = call "Options GFV.vi"("Anything"=w191, "error in (no error)"=w208, "Action(Get Settings)"=w179, "Setting ID"=Options_PageID."P 6 (Err)") -> ("error out"=w209:errorcluster)  [unwired: 13 in, 2 out]
                    n80 = call "Options GFV.vi"("Anything"=w192, "error in (no error)"=w209, "Action(Get Settings)"=w179, "Setting ID"=Options_PageID."P 5") -> ("error out"=w203:errorcluster)  [unwired: 13 in, 2 out]
                    n81 = call "Options GFV.vi"("Anything"=w193, "error in (no error)"=w203, "Action(Get Settings)"=w179, "Setting ID"=Options_PageID."P 4") -> ("error out"=w202:errorcluster)  [unwired: 13 in, 2 out]
                    n82 = call "Options GFV.vi"("Anything"=w194, "error in (no error)"=w202, "Action(Get Settings)"=w179, "Setting ID"=Options_PageID."P 3") -> ("error out"=w201:errorcluster)  [unwired: 13 in, 2 out]
                    n83 = call "Options GFV.vi"("Anything"=w195, "error in (no error)"=w201, "Action(Get Settings)"=w179, "Setting ID"=Options_PageID."P 2") -> ("error out"=w198:errorcluster)  [unwired: 13 in, 2 out]
                    n84 = call "Options GFV.vi"("Anything"=w196, "error in (no error)"=w198, "Action(Get Settings)"=w179, "Setting ID"=Options_PageID."P 1 (App)") -> ("error out"=w188:errorcluster)  [unwired: 13 in, 2 out]
                    n85 = call "Options GFV.vi"("Anything"=w186, "error in (no error)"=w188, "Action(Get Settings)"=w179, "Setting ID"=Options_PageID."C 1") -> ("error out"=w187:errorcluster)  [unwired: 13 in, 2 out]
                    n86 = call "Options GFV.vi"("Anything"=w185, "error in (no error)"=w187, "Action(Get Settings)"=w179, "Setting ID"=Options_PageID."C 2") -> ("error out"=w182:errorcluster)  [unwired: 13 in, 2 out]
                    n87 = call "Options GFV.vi"("error in (no error)"=w182, "Action(Get Settings)"=Action_GFV_Settings."Put In INI" ("Action")) -> ("error out"=w204:errorcluster)  [unwired: 15 in, 2 out]
                  }
                  frame True {
                    n88 = for {
                      shift-right: [w223] -> w215
                      shift-left: "" -> [w222]
                      tunnel: w213 -> [w220] mode=indexing
                      n89 = String Length(string=w220) -> (length=w221:i32)
                      n90 = case shown="1, Default" w221 {
                        tunnel: w222 -> [w224 w229]
                        tunnel: [w224 w226] -> w223
                        tunnel: w220 -> [_ w225]
                        frame 0 {
                        }
                        frame 1, Default {
                          n91 = Concatenate Strings(w229, "\r", "* " ("string"), w225) -> (w226:string)
                        }
                      }
                    }
                    n92 = Concatenate Strings("There is an issue with one or more options." ("message"), "\r", w215) -> (w214:string)
                    n93 = One Button Dialog(message=w214) -> ()  [unwired: 1 in, 1 out]
                  }
                }
              }
            }
          }
          event "Set current depth": Value Change {
            n94 = event-data() -> ()  [unwired: 1 in, 1 out]
            n95 = Bundle By Name(cluster=w232, "Depth Updated"=TRUE) -> (w231:T20)
          }
          event "Power Supply/PCP", "Modem Data", "Tractor Interface", "Modem Status": Value Change {
            n96 = event-data() -> ("OldVal"=w237:u16, "CtlRef"=w243:refnum<vi>, "NewVal"=w239:u16)  [unwired: 1 in]
            n97 = property class="Ring (strict)"(reference=w243) -> (reference out=w236:refnum<vi>, "Strings []"=w242:string[])  [unwired: 1 in, 1 out]
            n98 = Index Array(array=w242, index=w239) -> (element=w240:string)
            n99 = Equal?(x=w240, y="Refresh") -> (x = y?=w238:bool)
            n100 = case shown="True" w238 {
              tunnel: w245 -> [w254 w288]
              tunnel: [w253 w277] -> w244
              tunnel: w237 -> [_ w289]
              tunnel: w236 -> [_ w290]
              tunnel: w235 -> [_ w270]
              frame False {
                n101 = control-ref of="Power Supply/PCP"() -> (w249:refnum<vi>)
                n102 = control-ref of="Modem Data"() -> (w250:refnum<vi>)
                n103 = control-ref of="Tractor Interface"() -> (w251:refnum<vi>)
                n104 = control-ref of="Modem Status"() -> (w252:refnum<vi>)
                n105 = Build Array(w249, w250, w251, w252) -> (w248:refnum<vi>[])
                n106 = for {
                  tunnel: w248 -> [w265] mode=indexing
                  shift-right: [w264] -> w256
                  shift-left: w254 -> [w263]
                  tunnel: [w260] -> w258 mode=indexing
                  shift-right: [w262] -> w257
                  shift-left: i32[] [] -> [w261]
                  n107 = property class="Ring (strict)"(reference=w265, error in=w263) -> (error out=w264:errorcluster, "Value"=w260:u16)  [unwired: 1 out]
                  n108 = Greater Than 0?(x=w260) -> (x > 0?=w259:bool)
                  n109 = case shown="True" w259 {
                    tunnel: w260 -> [_ w269]
                    tunnel: [w266 w268] -> w262
                    tunnel: w261 -> [w266 w267]
                    frame False {
                    }
                    frame True {
                      n110 = Build Array (concatenate)(w267, w269) -> (w268:i32[])
                    }
                  }
                }
                n111 = call "Disable Ports already taken.vi"("error in (no error)"=w256, "Values"=w258, "COM Port numbers taken"=w257, "Ctrl References"=w248) -> ("error out"=w253:errorcluster)  [unwired: 7 in]
              }
              frame True {
                # "If refresh was selected the old value is written back to the control\nSince there is a chance that the list of COM port has changed the \nold selection are read out by name and not by value."
                n112 = property class="Ring (strict)"(reference=w290, error in=w288, "Value"=w289) -> (error out=w276:errorcluster)  [unwired: 1 out]
                n113 = control-ref of="Power Supply/PCP"() -> (w272:refnum<vi>)
                n114 = control-ref of="Modem Data"() -> (w273:refnum<vi>)
                n115 = control-ref of="Tractor Interface"() -> (w274:refnum<vi>)
                n116 = control-ref of="Modem Status"() -> (w275:refnum<vi>)
                n117 = Build Array(w272, w273, w274, w275) -> (w271:refnum<vi>[])
                n118 = call "Serial Port - Get Selected Names.vi"("error in (no error)"=w276, "Ctrl Refs in"=w271) -> ("error out"=w282:errorcluster, "Selected Names"=w287:string[])  [unwired: 8 in]
                n119 = call "Enumerer tilkoblede comporter.vi"("error in (no error)"=w282) -> ("Com port w Select string"=w281:string[], "error out"=w280:errorcluster)  [unwired: 11 in, 2 out]
                n120 = call "Serial Port - Append disconnected ports to list.vi"("error in (no error)"=w280, "Selected Values"=w270, "Connected COM Ports in"=w281) -> ("error out"=w284:errorcluster, "COM Ports out"=w283:string[])  [unwired: 7 in]
                n121 = call "Serial Port - Write Selected Names.vi"("error in (no error)"=w284, "Selected Names"=w287, "COM Port List"=w283, "Ctrl Refs in"=w271) -> ("error out"=w285:errorcluster, "Selected Values"=w278:i32[])  [unwired: 6 in]
                n122 = call "Serial Port - Find used serial ports.vi"("error in (no error)"=w285, "Selected Values"=w287, "COM Ports list"=w283) -> ("error out"=w286:errorcluster, "Items to disable"=w279:i32[])  [unwired: 7 in]
                n123 = call "Disable Ports already taken.vi"("error in (no error)"=w286, "Values"=w278, "COM Port numbers taken"=w279, "Ctrl References"=w271) -> ("error out"=w277:errorcluster)  [unwired: 7 in]
              }
            }
          }
          event "Cancel": Mouse Up {
            n124 = event-data() -> ()  [unwired: 1 in, 1 out]
          }
          event "Create system report": Mouse Up {
            n125 = event-data() -> ()  [unwired: 1 in, 1 out]
            n126 = call <vilib>:"Set Busy.vi"("error in (no error)"=w304) -> ("error out"=w302:errorcluster)  [unwired: 9 in, 1 out]
            n127 = local read "P 6 (Err)"() -> (w297:T13)
            n128 = call "emi_Get system Info.vi"("error in (no error)"=w302) -> ("Info retreived"=w299:bool, "System Info"=w298:string, "error out"=w301:errorcluster)  [unwired: 12 in]
            n129 = case shown="True" w299 {
              tunnel: w301 -> [w307 w310]
              tunnel: [w307 w324] -> w300
              tunnel: w298 -> [_ w322]
              tunnel: w297 -> [_ w332]
              frame False {
                n130 = One Button Dialog(message="There was a problem retreiving system information. No report genereated") -> ()  [unwired: 1 in, 1 out]
              }
              frame True {
                # "TODO:_ create report File. Prompt for location"
                n131 = Unbundle By Name(w332) -> ("Error and event files"=w331:path)
                n132 = Get Date/Time In Seconds() -> (seconds since 1Jan1904=w323:timestamp)
                n133 = Format Date/Time String(time format string (%c)="%Y%m%d %H%M%S", seconds (now)=w323) -> (date/time string=w329:string)  [unwired: 1 in]
                n134 = Concatenate Strings(w329, ".sysrep.txt") -> (w327:string)
                n135 = Build Path(base path=w331, name or relative path=w327) -> (appended path=w312:path)
                n136 = call "emi_Check-Create Folders in path.vi"("Path including file"=w312, "error in (no error)"=w310) -> ("Path out"=w309:path, "error out"=w311:errorcluster)  [unwired: 11 in, 1 out]
                n137 = Open/Create/Replace File(file path (use dialog)=w309, error in=w311, operation (0:open)=T27."replace or create", access (0:read/write)=enum16{"read/write", "read-only", "write-only"}."write-only") -> (refnum out=w316:refnum<file>, error out=w321:errorcluster)  [unwired: 2 in, 1 out]
                n138 = Set File Position(refnum=w316, from (0:start)=enum16{"start", "end", "current"}."start", error in=w321) -> (refnum out=w315:refnum<file>, error out=w320:errorcluster)  [unwired: 1 in]
                n139 = Write to Text File(file (use dialog)=w315, text=w322, error in=w320) -> (refnum out=w314:refnum<file>, error out=w318:errorcluster)  [unwired: 1 in, 1 out]
                n140 = Close File(refnum=w314, error in=w318) -> (error out=w317:errorcluster)  [unwired: 1 out]
                n141 = Path To String(path=w309) -> (string=w308:string)
                n142 = case shown="Error" w317 {
                  selector: w317 -> [w336 w338]
                  tunnel: [w336 w338] -> w313
                  tunnel: w308 -> [w333 _]
                  frame No Error {
                    n143 = Concatenate Strings("System report created: " ("message"), w333) -> (w334:string)
                    n144 = One Button Dialog(message=w334) -> ()  [unwired: 1 in, 1 out]
                  }
                  frame Error {
                    n145 = One Button Dialog(message="System report could not be generated") -> ()  [unwired: 1 in, 1 out]
                  }
                }
                n146 = call <vilib>:"Clear Errors.vi"("error in (no error)"=w313) -> ("error out"=w324:errorcluster)  [unwired: 6 in]
              }
            }
            n147 = call <vilib>:"Unset Busy.vi"("error in (no error)"=w300) -> ("error out"=w303:errorcluster)  [unwired: 10 in]
          }
          event "Help": Value Change {
            n148 = event-data() -> ()  [unwired: 1 in, 1 out]
            n149 = case shown="True" "Help" {
              tunnel: [w345 w356] -> w341
              tunnel: w340 -> [w345 w354]
              frame False {
              }
              frame True {
                n150 = local read "Tab Control"() -> (w355:T1)
                n151 = Format Into String(format string="%s", initial string="Options", error in=w354, w355) -> (resulting string=w348:string, error out=w351:errorcluster)
                n152 = Search and Replace String(replace all?=TRUE ("replace all? (F)"), input string=w348, search string=" ", error in=w351) -> (result string=w346:string, error out=w350:errorcluster)  [unwired: 4 in, 2 out]
                n153 = call "Open App Help file.vi"("Help Tag (\"\")"=w346, "error In"=w350) -> ("error out"=w356:errorcluster)  [unwired: 13 in]
              }
            }
          }
        }
      }
    }
    frame Error {
      w357 = FALSE
      n154 = Unbundle(w363) -> ("code"=w360:i32, "source"=w359:string)  [unwired: 1 out]
      n155 = Format Into String(format string="%d    %s", initial string="Options dialog could not be displayed due to error\n\nMake sure that the the Visa libray from NI is installed." ("message"), w360, w359) -> (resulting string=w361:string)  [unwired: 1 in, 1 out]
      n156 = One Button Dialog(message=w361) -> ()  [unwired: 1 in, 1 out]
    }
  }
  "OK" <- w8
  "Restart software" <- w1
  n157 = call "emi_Dialog End.vi"("error in"=w7) -> ("error out"=→"error out":errorcluster)  [unwired: 14 in]
